vi "两片74HC162设计一个二十四进制计数器.vi"() -> ()   [LabVIEW 2018]
panel:
  in  "确定按钮":bool
  out "H10-1":bool
  out "H10-2":bool
  out "L10-1":bool
  out "L10-2":bool
  out "L10-3":bool
  out "L10-4":bool
  in  "CLK":bool
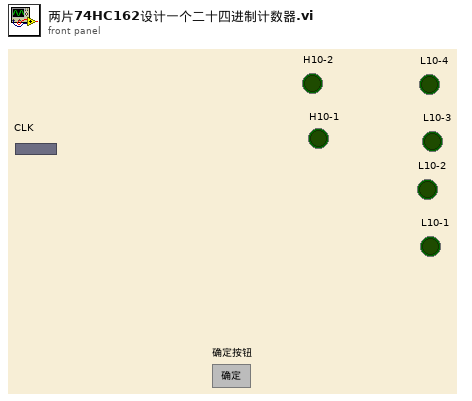
[diagram p1: front panel]
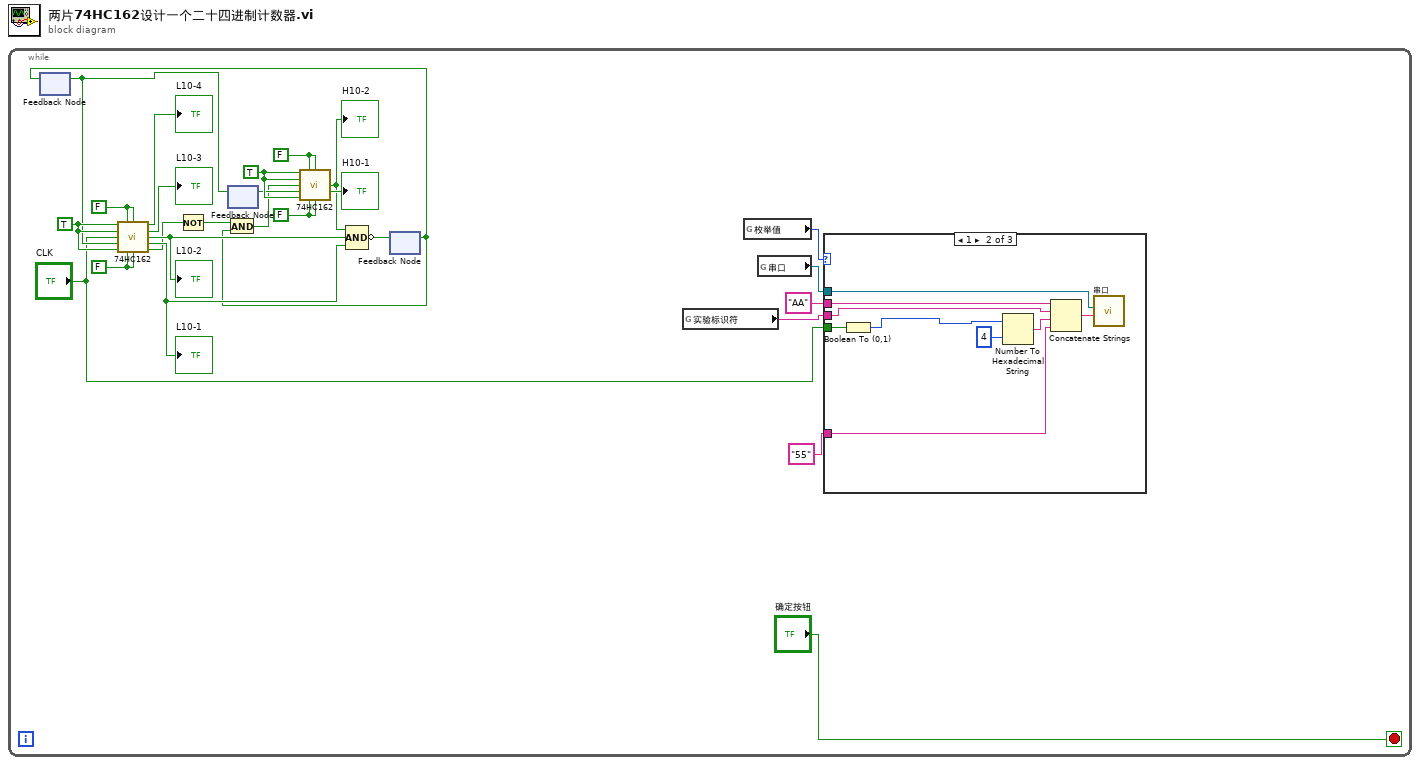
[diagram p0: block diagram]
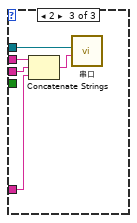
[diagram p3: hidden frame]
diagram:
  n1 = while {
    stop <- "确定按钮" stop-if-true
    w19 = FALSE
    w20 = FALSE
    w21 = FALSE
    w22 = FALSE
    w23 = TRUE
    w26 = TRUE
    n2 = feedback #1() -> (w13:bool)  [unwired: 1 in]
    n3 = call "74HC162.vi"("EP"=w26, "D2"=w22, "D3"=w22, "ET"=w26, "cp"="CLK", "CR`"=w13, "LD`"=w26, "D1"=w21, "D0"=w21) -> ("Q3"=→"L10-4":bool, "Q2"=→"L10-3":bool, "Q1"=w16:bool, "Q0"=w15:bool, "RCO"=w12:bool)  [unwired: 2 in]
    "L10-2" <- w16
    "L10-1" <- w15
    n4 = Not(x=w12) -> (.not. x?=w11:bool)
    n5 = feedback #2() -> (w14:bool)  [unwired: 1 in]
    n6 = feedback-in #2(w13) -> ()
    n7 = feedback #3() -> (w8:bool)  [unwired: 1 in]
    n8 = feedback-in #1(w8) -> ()
    n9 = And(x=w11, y=w8) -> (x .and. y?=w10:bool)
    n10 = call "74HC162.vi"("EP"=w23, "D2"=w20, "D3"=w20, "ET"=w23, "cp"=w10, "CR`"=w14, "LD`"=w23, "D1"=w19, "D0"=w19) -> ("Q1"=w17:bool, "Q0"=→"H10-1":bool)  [unwired: 2 in, 3 out]
    "H10-2" <- w17
    n11 = Compound Arithmetic op=AND ("复合运算")(w17, w16, w15) -> (invert w9:bool)
    n12 = feedback-in #3(w9) -> ()
    n13 = global read "全局变量.vi" "实验标识符"() -> (w4:string)
    n14 = global read "全局变量.vi" "枚举值"() -> (w6:i8)
    n15 = global read "全局变量.vi" "串口"() -> (w5:refnum<visa-resource-name>)
    n16 = case shown="1" w6 {
      tunnel: w5 -> [_ w34 w38]
      tunnel: w4 -> [_ w33 w39]
      tunnel: "55" -> [_ w32 w36]
      tunnel: "AA" -> [_ w31 w37]
      tunnel: "CLK" -> [_ w27 _]
      frame 0, Default {
      }
      frame 1 {
        n17 = Boolean To (0,1)(Boolean=w27) -> (0, 1=w28:i16)
        n18 = Number To Hexadecimal String(1:4, 2:w28) -> (0:w29:string)
        n19 = Concatenate Strings(w31, w33, w29, w32) -> (w35:string)
        n20 = call "串口.vi"("字符串"=w35, "VISA resource name"=w34) -> ()  [unwired: 10 in]
      }
      frame 2 {
        n21 = Concatenate Strings(w37, w39, w36) -> (w40:string)
        n22 = call "串口.vi"("字符串"=w40, "VISA resource name"=w38) -> ()  [unwired: 10 in]
      }
    }
  }
